vi "Consumer.vi"(8 "error in (no error)":errorcluster, 9 "Data":variant, 10 "Case ID":string, 11 "uService Test in":refnum<class "test_us.lvclass">) -> (0 "error out":errorcluster, 3 "uService Test out":refnum<class "test_us.lvclass">)   [LabVIEW 2026, in "test_us.lvlib" / "test_us.lvclass"]
uses:
  test_us.lvclass
  C:/LabVIEW Code/TALOS/talos/Father of all uServices/Father of all uServices/Father of all uServices.lvclass
  Test uS Consumer case selector.ctl
  Father of all uServices/Father of all uServices/Father of all uServices.lvclass/Father of all uServices.ctl
  Ancestor/Ancestor/Ancestor.lvclass/Ancestor.ctl
  Ancestor/Ancestor/Infinite Message Selector.ctl
  Support VIs/Substitute Error.vi
  Support VIs/Generate Error.vi
  FGV/Error Memory/Get Error Description.vi
  Support VIs/Get PC name.vi
  Ancestor/Ancestor/Read ID.vi
  Support VIs/Get Class Name.vi
  <vilib>/Utility/error.llb/Clear Errors.vi
  FGV/Error Memory/Error Memory Core.vi
  <vilib>/AdvancedString/Delimited String to 1D String Array.vi
  <vilib>/AdvancedString/Delimited String to 1D String Array (string).vi
  Support VIs/Circus Root Path.vi
  FGV/Error Memory/Error Crt Lvl checker.vi
  FGV/Error Memory/Error Memory Core.vi/40c8088d-b597-4017-91af-faa98e00292e.vi
  FGV/Error Memory/Error Memory Core.vi/d4a3ab98-063c-4e44-b43d-fbdcfe6c2be2.vi
  Support VIs/Global Memory.vi
  <vilib>/Utility/LVClass/Get LV Class Name.vi
  Support VIs/Is in Packed Library.vi
  Support VIs/TALOS Root path.vi
  Support VIs/Read CSV worksheet.vi
  Support VIs/Global Constants.vi
  <vilib>/Utility/error.llb/General Error Handler.vi
  Support VIs/Error Log.vi
  Ancestor/Ancestor/Ancestor.lvclass
  <vilib>/Comparison/Equal/Equal Functor/Equal Functor.lvclass
  Father of all uServices/Father of all uServices/Father of all uServices.lvclass
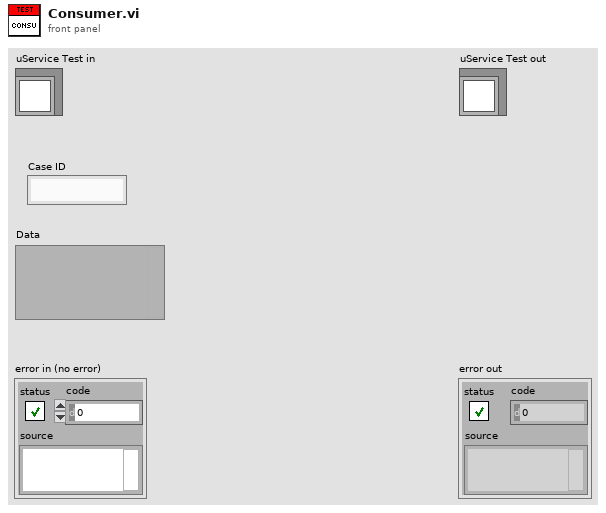
[diagram p1: front panel]
types:
  T1 = typedef "test_us.lvlib/test_us.lvclass/Test uS Consumer case selector.ctl" = enum16{"graph", "infinite", "Start infinite", "Check infinite", "Stop infinite", "Delayed message"}
  T2 = typedef "TALOS.lvlib/Ancestor.lvlib/Ancestor.lvclass/Infinite Message Selector.ctl" = enum16{"Start", "Stop", "Check", "Flush (Stop all)", "Init"}
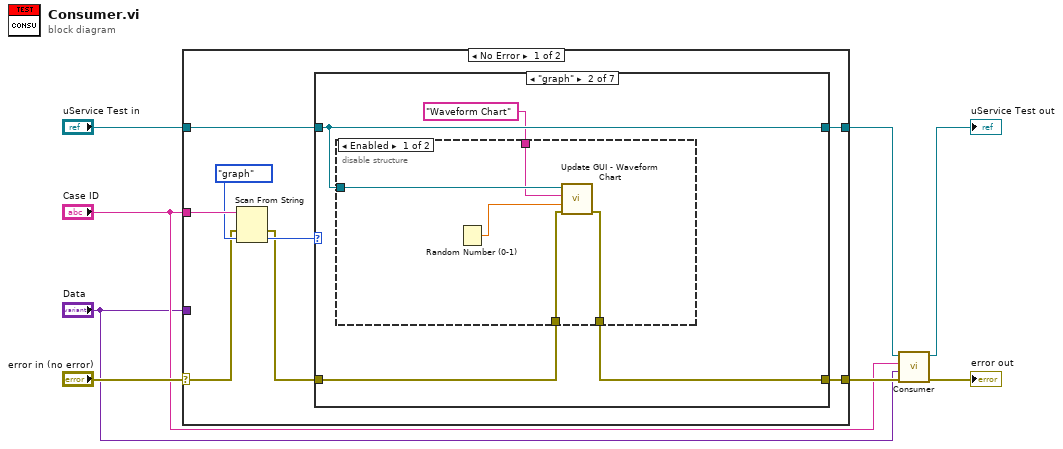
[diagram p0: block diagram]
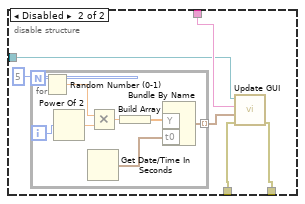
[diagram p3: hidden frame]
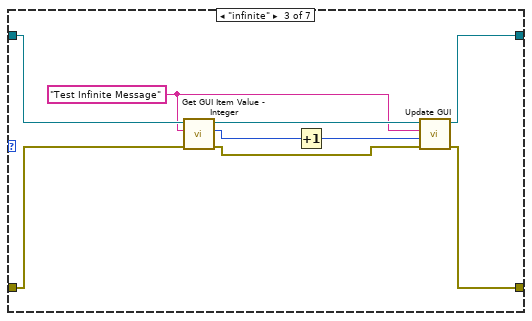
[diagram p4: hidden frame]
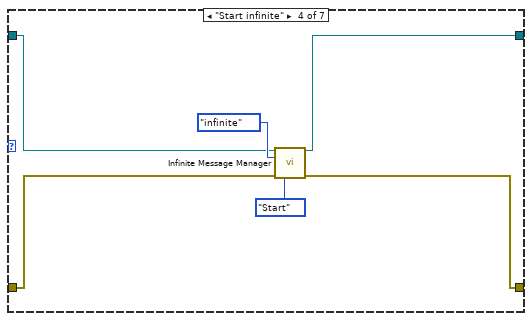
[diagram p5: hidden frame]
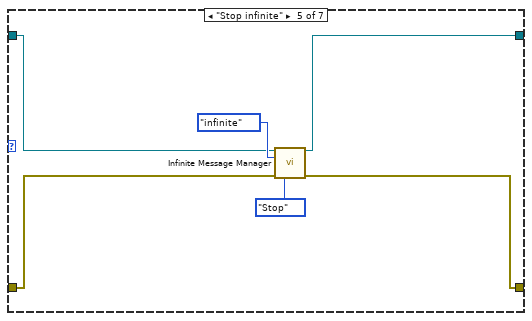
[diagram p6: hidden frame]
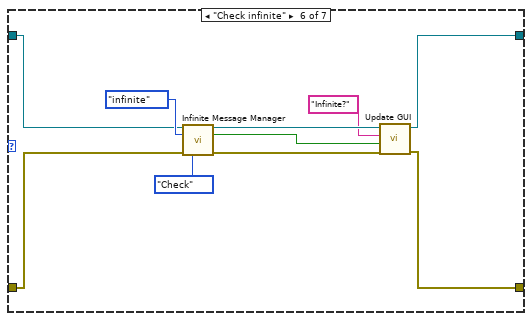
[diagram p7: hidden frame]
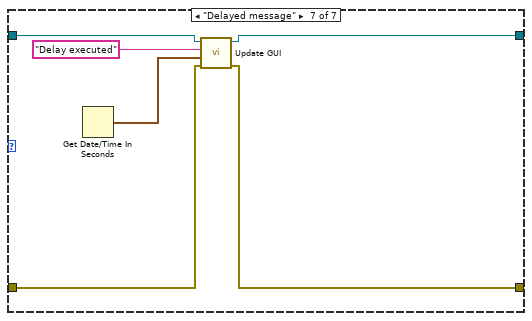
[diagram p8: hidden frame]
diagram:
  n1 = case shown="No Error" "error in (no error)" {
    selector: "error in (no error)" -> [w10 w78]
    tunnel: [w15 w79] -> w3
    tunnel: "uService Test in" -> [w16 w79]
    tunnel: [w14 w78] -> w6
    tunnel: "Case ID" -> [w13 _]
    tunnel: "Data" -> [_ _]
    frame No Error {
      n2 = Scan From String(input string=w13, error in=w10, default 1=Test_uS_Consumer_case_selector."graph" ("arsnars consumer case selector")) -> (error out=w9:errorcluster, output 1=w11:T1)  [unwired: 2 in, 2 out]
      n3 = case shown="\"graph\"" w11 {
        tunnel: w16 -> [w18 w22 w48 w53 w59 w65 w77]
        tunnel: [w18 w22 w42 w52 w58 w64 w76] -> w15
        tunnel: [w17 w21 w41 w50 w56 w62 w74] -> w14
        tunnel: w9 -> [w17 w20 w46 w51 w57 w63 w75]
        frame Default {
        }
        frame "graph" {
          n4 = disable-structure shown="Enabled" {
            disable-tunnel: w22 -> [w27 w29]
            disable-tunnel: [w26 w31] -> w21
            disable-tunnel: w20 -> [w25 w32]
            disable-tunnel: "Waveform Chart" ("GUI Item Name") -> [w23 w30]
            frame Enabled {
              n5 = Random Number (0-1)() -> (number: 0 to 1=w24:dbl)
              n6 = call "Update GUI - Waveform Chart.vi"("error in (no error)"=w25, "Point value"=w24, "GUI Item Name"=w23, "uService Template in"=w27) -> ("error out"=w26:errorcluster)  [unwired: 6 in, 1 out]
            }
            frame Disabled {
              n7 = for {
                N: 5 -> [_]
                tunnel: [w39] -> w28 mode=indexing
                i -> [w35]
                n8 = Random Number (0-1)() -> (number: 0 to 1=w37:dbl)
                n9 = Power Of 2(x=w35) -> (2^x=w36:dbl)
                n10 = Get Date/Time In Seconds() -> (seconds since 1Jan1904=w40:timestamp)
                n11 = Multiply(x=w37, y=w36) -> (x*y=w34:dbl)
                n12 = Build Array(w34) -> (w38:dbl[])
                n13 = Bundle By Name("Y"=w38, "t0"=w40) -> (w39:waveform(dbl))  [unwired: 1 in]
              }
              n14 = call "Update GUI.vi"("error in (no error)"=w32, "Data"=w28, "GUI Item Name"=w30, "uService Template in"=w29) -> ("error out"=w31:errorcluster)  [unwired: 6 in, 1 out]
            }
          }
        }
        frame "infinite" {
          w47 = "Test Infinite Message" ("GUI Item Name")
          n15 = call "Get GUI Item Value - Integer.vi"("error in (no error)"=w46, "FP Item Name"=w47, "uService Template in"=w48) -> ("error out"=w43:errorcluster, "Value"=w45:i32, "uService Template out"=w49:refnum<class "test_us.lvclass">)  [unwired: 6 in]
          n16 = Increment(x=w45) -> (x+1=w44:i32)
          n17 = call "Update GUI.vi"("error in (no error)"=w43, "Data"=w44, "GUI Item Name"=w47, "uService Template in"=w49) -> ("error out"=w41:errorcluster, "uService Template out"=w42:refnum<class "test_us.lvclass">)  [unwired: 6 in]
        }
        frame "Start infinite" {
          n18 = call-dynamic "Infinite Message Manager.vi"("Father of all uServices in"=w53, "Consumer Case Selector"=Test_uS_Consumer_case_selector."infinite" ("arsnars consumer case selector"), "error in (no error)"=w51, "Infinite Message Selector"=Infinite_Message_Selector."Start") -> ("Father of all uServices out"=w52:refnum<class "test_us.lvclass">, "error out"=w50:errorcluster)  [unwired: 9 in, 1 out]
        }
        frame "Stop infinite" {
          n19 = call-dynamic "Infinite Message Manager.vi"("Father of all uServices in"=w59, "Consumer Case Selector"=Test_uS_Consumer_case_selector."infinite" ("arsnars consumer case selector"), "error in (no error)"=w57, "Infinite Message Selector"=Infinite_Message_Selector."Stop") -> ("Father of all uServices out"=w58:refnum<class "test_us.lvclass">, "error out"=w56:errorcluster)  [unwired: 9 in, 1 out]
        }
        frame "Check infinite" {
          n20 = call-dynamic "Infinite Message Manager.vi"("Father of all uServices in"=w65, "Consumer Case Selector"=Test_uS_Consumer_case_selector."infinite" ("arsnars consumer case selector"), "error in (no error)"=w63, "Infinite Message Selector"=Infinite_Message_Selector."Check") -> ("Father of all uServices out"=w69:refnum<class "test_us.lvclass">, "Exists?"=w66:bool, "error out"=w67:errorcluster)  [unwired: 9 in]
          n21 = call "Update GUI.vi"("error in (no error)"=w67, "Data"=w66, "GUI Item Name"="Infinite?", "uService Template in"=w69) -> ("error out"=w62:errorcluster, "uService Template out"=w64:refnum<class "test_us.lvclass">)  [unwired: 6 in]
        }
        frame "Delayed message" {
          n22 = Get Date/Time In Seconds() -> (seconds since 1Jan1904=w72:timestamp)
          n23 = call "Update GUI.vi"("error in (no error)"=w75, "Data"=w72, "GUI Item Name"="Delay executed", "uService Template in"=w77) -> ("error out"=w74:errorcluster, "uService Template out"=w76:refnum<class "test_us.lvclass">)  [unwired: 6 in]
        }
      }
    }
    frame Error {
    }
  }
  n24 = call-parent "Consumer.vi"("error in (no error)"=w6, "Data"="Data", "Case ID"="Case ID", "uService Template in"=w3) -> ("error out"=→"error out":errorcluster, "uService Template out"=→"uService Test out":refnum<class "test_us.lvclass">)  [unwired: 6 in]
